vi "XIPIN_AXI_Video_Direct_Memory_Access_6_2.vi"   [LabVIEW 2017]
doc: "The Xilinx AXI Video DMA LogiCORE provides a flexible interface for controlling and synchronizing video frame buffers from external memory. Multiple VDMAs from different clock domains can be linked together to control frame buffer reads and writes from multiple sources. Automatic frame skips and repeats are performed to seamlessly allow frame rate conversion. Support for up to 32 external frame buffers with image sizes of 4k x4k is provided. The core is programmable through a comprehensive register interface for setting and controlling frame synchronization (can be turned on/off in real-time), frame read/write delays, source synchronization switching, circular buffer enable and more using logic or a microprocessor.Error interrupt status bits provided for processor monitoring.\n------------------------------------\n<b>Need License</b> : No\n<b>Interface</b> : AXI4 AXI4-Stream"
uses:
  <vilib>/rvi/XilinxIP/XIPIN_XNode/niFpgaXIPIN.xnode
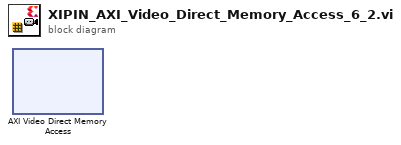
[diagram p0: block diagram]
diagram:
  n1 = xnode ("AXI Video Direct Memory Access")() -> ()
